vi "Test Worker Handle Job.vi"(8 "error in (no error)":errorcluster, 11 "Worker Test in":refnum<class "Worker Test.lvclass">) -> (0 "error out":errorcluster, 3 "Worker Test out":refnum<class "Worker Test.lvclass">)   [LabVIEW 2020, in "Worker Test.lvclass"]
uses:
  Worker Test.lvclass
  C:/Program Files (x86)/National Instruments/LabVIEW 2020/vi.lib/Asteme/LUnit/Test Case.lvclass
  Worker/Worker.lvclass
  C:/Program Files (x86)/National Instruments/LabVIEW 2020/vi.lib/Asteme/Triarc Framework/Process/Process.lvclass
  <vilib>/Asteme/Triarc Framework Test Suite/Mock Error Handler/Mock Error Handler.lvclass
  C:/Program Files (x86)/National Instruments/LabVIEW 2020/vi.lib/Asteme/Triarc Framework/Error Handler Interface/Error Handler Interface.lvclass
  <vilib>/Asteme/Triarc Framework/Process/Process.lvclass/Process.ctl
  <vilib>/Asteme/LUnit/Test Case.lvclass/Test Case.ctl
  <vilib>/Asteme/LUnit/LUnit Assertion Result.lvclass/LUnit Assertion Result.ctl
  <vilib>/Asteme/Triarc Framework/Process/Protected/Messaging/Enqueue Message.vi
  <vilib>/Asteme/Triarc Framework/Process/Public/Lifecycle/Get Lifecycle State.vi
  <vilib>/Asteme/Triarc Framework/Process/Private/SubVIs/Wait for finish.vi
  <vilib>/Asteme/Triarc Framework/Process/Private/SubVIs/Set Lifecycle State.vi
  <vilib>/Asteme/LUnit/Palette/Fail.vi
  <vilib>/Asteme/LUnit/Palette/Pass.vi
  <vilib>/Asteme/LUnit/Variant to string.vi
  <vilib>/Asteme/LUnit/Set Assertion Type.vi
  <vilib>/Asteme/LUnit/Add test result.vi
  <vilib>/Asteme/LUnit/LUnit Get Test Case.vi
  <vilib>/Asteme/LUnit/Assertion Result/LUnit Get Test Name.vi
  <vilib>/Asteme/LUnit/LUnit Write Message.vi
  <vilib>/Asteme/LUnit/LUnit Write Description.vi
  <vilib>/Asteme/LUnit/LUnit Write Skipped.vi
  <vilib>/Utility/error.llb/Clear Errors.vi
  <vilib>/Asteme/LUnit/LUnit Write Passed.vi
  <vilib>/Asteme/LUnit/LUnit Write Assertion Type.vi
  <vilib>/Asteme/LUnit/Read Test Case Name.vi
  <vilib>/Utility/error.llb/Error Cluster From Error Code.vi
  <vilib>/Utility/Data Type/Get Type Information.vi
  <vilib>/Utility/LVClass/Get LV Class Name.vi
  <vilib>/Asteme/LUnit/LUnit Assertion Result.lvclass
  <vilib>/Asteme/Triarc Framework/Process/Process.lvclass
  <vilib>/Asteme/LUnit/Test Case.lvclass
  C:/Users/anton/Documents/GitHub/Triarc-Examples/Coffee Shop/Person/Person.lvclass
  C:/Program Files (x86)/National Instruments/LabVIEW 2020/vi.lib/Asteme/Triarc Framework/View/View.lvclass
  C:/Program Files (x86)/National Instruments/LabVIEW 2020/vi.lib/Asteme/Triarc Framework/Base/Base.lvclass
  C:/Program Files (x86)/National Instruments/LabVIEW 2020/vi.lib/Asteme/Triarc Framework/Logging/Logging.lvclass
  C:/Users/anton/Documents/GitHub/Triarc-Examples/Coffee Shop/Worker/Worker.lvclass
  C:/Users/anton/Documents/GitHub/Triarc-Examples/Coffee Shop/Person Test/Person Test.lvclass
  C:/Program Files (x86)/National Instruments/LabVIEW 2020/vi.lib/Asteme/Triarc Framework Test Suite/View Test/View Test.lvclass
  C:/Program Files (x86)/National Instruments/LabVIEW 2020/vi.lib/Asteme/Triarc Framework Test Suite/Process Test/Process Test.lvclass
  C:/Program Files (x86)/National Instruments/LabVIEW 2020/vi.lib/Asteme/Triarc Framework Test Suite/Base Class Test/Base Test.lvclass
  C:/Users/anton/Documents/GitHub/Triarc-Examples/Coffee Shop/Worker Test/Worker Test.lvclass
  C:/Program Files (x86)/National Instruments/LabVIEW 2020/vi.lib/Asteme/Triarc Framework Test Suite/Mock Error Handler/Mock Error Handler.lvclass
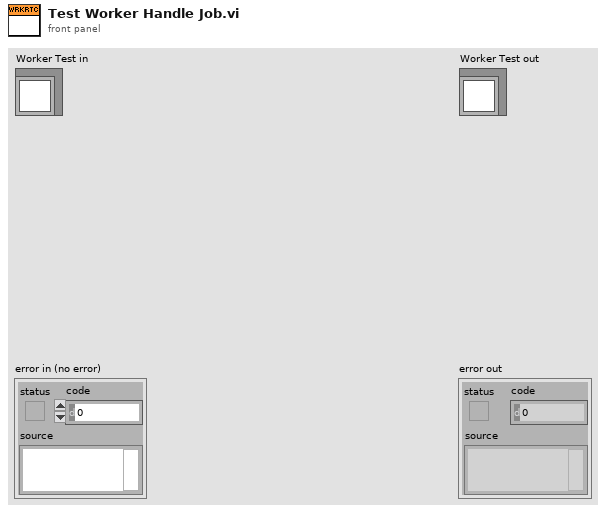
[diagram p1: front panel]
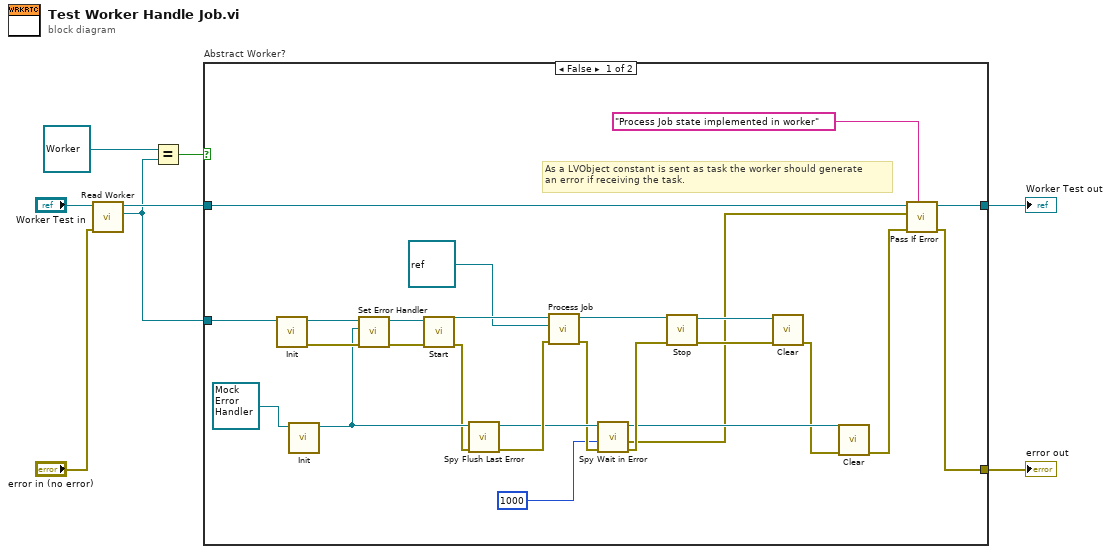
[diagram p0: block diagram]
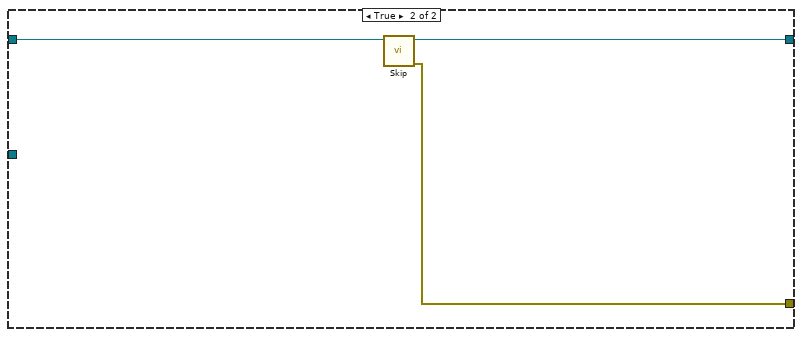
[diagram p2: hidden frame]
diagram:
  n1 = call "Read Worker.vi"("error in (no error)"="error in (no error)", "Worker Test in"="Worker Test in") -> ("Worker"=w2:refnum<class "Worker.lvclass">, "Worker Test out"=w5:refnum<class "Worker Test.lvclass">)  [unwired: 7 in, 1 out]
  n2 = Equal?(x=refnum<class "Worker.lvclass"> refnum ("Worker"), y=w2) -> (x = y?=w1:bool)
  n3 = case "Abstract Worker?" shown="False" w1 {
    tunnel: [w14 w35] -> w6
    tunnel: w5 -> [w13 w37]
    tunnel: [w12 w36] -> w4
    tunnel: w2 -> [w10 _]
    frame False {
      # "As a LVObject constant is sent as task the worker should generate \nan error if receiving the task."
      n4 = call-dynamic "Init.vi"("View In"=w10) -> ("error out"=w34:errorcluster, "View Out"=w30:refnum<class "Worker.lvclass">)  [unwired: 9 in]
      n5 = call-dynamic "Init.vi"("Mock Error Handler In"=refnum<class "Mock Error Handler.lvclass"> refnum) -> ("Mock Error Handler Out"=w27:refnum<class "Mock Error Handler.lvclass">)  [unwired: 9 in, 1 out]
      n6 = call <vilib>:"Set Error Handler.vi"("error in (no error)"=w34, "Error Handler"=w27, "Process In"=w30) -> ("error out"=w31:errorcluster, "Process Out"=w29:refnum<class "Worker.lvclass">)  [unwired: 7 in]
      n7 = call <vilib>:"Start.vi"("error in (no error)"=w31, "Process In"=w29) -> ("error out"=w26:errorcluster, "Process Out"=w25:refnum<class "Worker.lvclass">)  [unwired: 8 in]
      n8 = call <vilib>:"Spy Flush Last Error.vi"("error in (no error)"=w26, "Mock Error Handler In"=w27) -> ("error out"=w24:errorcluster, "Mock Error Handler Out"=w21:refnum<class "Mock Error Handler.lvclass">)  [unwired: 7 in, 1 out]
      n9 = call "Process Job.vi"("error in (no error)"=w24, "Task"=refnum<class> refnum, "Worker In"=w25) -> ("error out"=w20:errorcluster, "Worker Out"=w22:refnum<class "Worker.lvclass">)  [unwired: 7 in]
      n10 = call <vilib>:"Spy Wait in Error.vi"("error in (no error)"=w20, "timeout in ms (-1)"=1000, "Mock Error Handler In"=w21) -> ("error out"=w19:errorcluster, "Errors"=w9:errorcluster, "Mock Error Handler Out"=w18:refnum<class "Mock Error Handler.lvclass">)  [unwired: 4 in, 2 out]
      n11 = call <vilib>:"Stop.vi"("error in (no error)"=w19, "Process In"=w22) -> ("error out"=w32:errorcluster, "Process Out"=w33:refnum<class "Worker.lvclass">)  [unwired: 7 in, 1 out]
      n12 = call-dynamic "Clear.vi"("error in (no error)"=w32, "View In"=w33) -> ("error out"=w17:errorcluster)  [unwired: 9 in]
      n13 = call-dynamic "Clear.vi"("error in (no error)"=w17, "Mock Process In"=w18) -> ("error out"=w16:errorcluster)  [unwired: 9 in]
      n14 = call <vilib>:"Pass If Error.vi"("Description"="Process Job state implemented in worker", "error in (no error)"=w16, "Assert error"=w9, "Test Case In"=w13) -> ("error out"=w14:errorcluster, "Test Case Out"=w12:refnum<class "Worker Test.lvclass">)  [unwired: 6 in]
    }
    frame True {
      n15 = call <vilib>:"Skip.vi"("Test Case In"=w37) -> ("error out"=w35:errorcluster, "Test Case Out"=w36:refnum<class "Worker Test.lvclass">)  [unwired: 9 in]
    }
  }
  "error out" <- w6
  "Worker Test out" <- w4
